vi "Create Waveform.vi"(5 "Unit":string="NI_ChannelName", 6 "dt":dbl, 7 "Channel name":string="NI_ChannelName", 8 "error in (no error)":errorcluster, 9 "t0":timestamp, 10 "index":i32, 11 "array":dbl[](array[numeric])) -> (0 "error out":errorcluster, 2 "Value":dbl, 3 "output waveform":waveform(dbl))   [LabVIEW 2019]
doc: "This example performs a serial port write and a serial port read. The parameters set for the serial port must match the parameters of the connected instrument or device. The VISA Configure Serial Port VI sets the configuration parameters. The front panel displays the controls used to configure the basic parameters, such as baud rate, data bits, and parity. The VI passes the VISA resource name to other VIs that perform operations on that VISA resource. The VISA Write function sends a command to the serial device and the VISA Read function returns data based on the command. The VISA Close function then closes the reference to the serial device. It is important to close the reference; otherwise, further communication through that port might not be possible."
panel:
  # "Create Waveform"
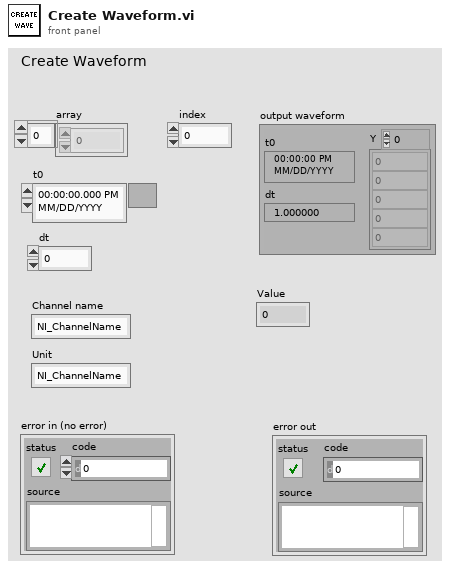
[diagram p1: front panel]
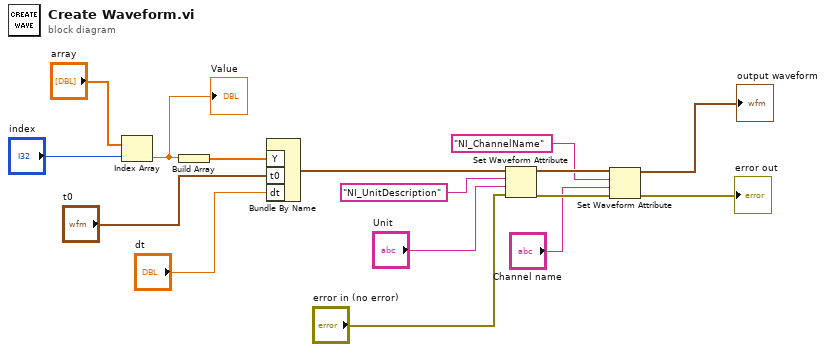
[diagram p0: block diagram]
diagram:
  n1 = Index Array(array="array", index="index") -> (element=w15:dbl)
  "Value" <- w15
  n2 = Build Array(w15) -> (w14:dbl[])
  n3 = Bundle By Name("Y"=w14, "t0"="t0", "dt"="dt") -> (w13:waveform(dbl))  [unwired: 1 in]
  n4 = Set Waveform Attribute(4:"error in (no error)", 5:"Unit", 6:"NI_UnitDescription", 7:w13) -> (0:w8:errorcluster, 3:w11:waveform(dbl))  [unwired: 1 out]
  n5 = Set Waveform Attribute(4:w8, 5:"Channel name", 6:"NI_ChannelName" ("name"), 7:w11) -> (0:→"error out":errorcluster, 3:→"output waveform":waveform(dbl))  [unwired: 1 out]
